vi "S2C_Access_ReadDrvCfg.vi"(8 "Error In":errorcluster) -> (0 "Error Out":errorcluster)   [LabVIEW 2015]
doc: "Reads the data contained within the Settings file and loads the data into VI specific global variables."
uses:
  Core/Command/S2C_CMD_Globals.vi
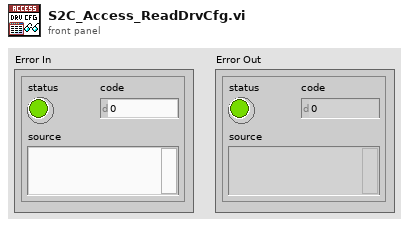
[diagram p1: front panel]
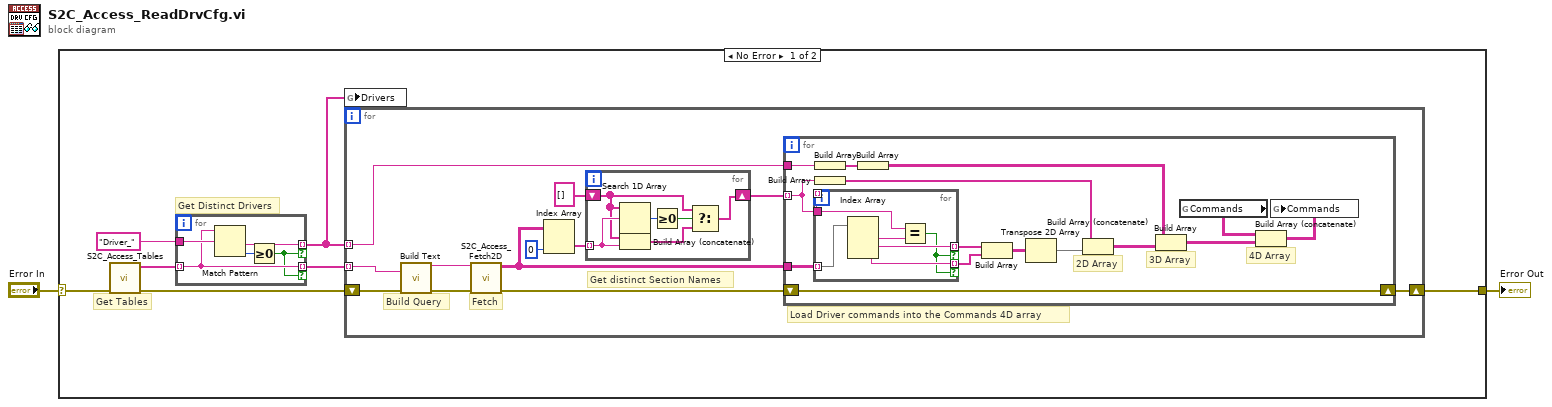
[diagram p0: block diagram]
diagram:
  n1 = case shown="No Error" "Error In" {
    selector: "Error In" -> [w5 w54]
    tunnel: [w4 w54] -> w1
    frame No Error {
      # "Get Distinct Drivers"
      # "Get Tables"
      n2 = call "S2C_Access_Tables.vi"("Error In"=w5) -> ("Error Out"=w7:errorcluster, "Tables"=w9:string[])  [unwired: 9 in]
      n3 = for {
        tunnel: w9 -> [w51] mode=indexing
        tunnel: "Driver_" -> [w53]
        tunnel: [w51] -> w6 mode=indexing if=w49
        tunnel: [w50] -> w3 mode=indexing if=w49
        n4 = Match Pattern(string=w51, regular expression=w53) -> (after substring=w50:string, offset past match=w52:i32)  [unwired: 1 in, 2 out]
        n5 = Greater Or Equal To 0?(x=w52) -> (x >= 0?=w49:bool)
      }
      n6 = global write "S2C_CMD_Globals.vi" "Drivers"(w3) -> ()
      n7 = for {
        shift-right: [w11] -> w4
        shift-left: w7 -> [w21]
        tunnel: w6 -> [w15] mode=indexing
        tunnel: w3 -> [w10] mode=indexing
        # "Load Driver commands into the Commands 4D array"
        # "Get distinct Section Names"
        # "Fetch"
        # "Build Query"
        n8 = call "Build Text"("Driver"=w15, "error in (no error)"=w21) -> ("Result"=w19:string, "error out"=w20:errorcluster)  [unwired: 12 in]
        n9 = call "S2C_Access_Fetch2D.vi"("Error In"=w20, "Query"=w19) -> ("Error Out"=w14:errorcluster, "Data"=w13:string[][])  [unwired: 8 in]
        n10 = Index Array(array=w13, index (col)=0 ("disabled index (col)")) -> (element=w17:string[])  [unwired: 1 in]
        n11 = for {
          shift-right: [w43] -> w12
          shift-left: string[] [] -> [w45]
          tunnel: w17 -> [w46] mode=indexing
          n12 = Search 1D Array(1D array=w45, element=w46) -> (index of element=w48:i32)  [unwired: 1 in]
          n13 = Build Array (concatenate)(w45, w46) -> (w44:string[])
          n14 = Greater Or Equal To 0?(x=w48) -> (x >= 0?=w47:bool)
          n15 = Select(t=w45, s=w47, f=w44) -> (s? t:f=w43:string[])
        }
        n16 = for {
          tunnel: w13 -> [w36]
          shift-right: [w35] -> w11
          shift-left: w14 -> [w35]
          tunnel: w12 -> [w32] mode=indexing
          tunnel: w10 -> [w34]
          # "2D Array"
          # "3D Array"
          # "4D Array"
          n17 = for {
            tunnel: w36 -> [w42] mode=indexing
            tunnel: [w40] -> w31 mode=indexing if=w38
            tunnel: [w39] -> w30 mode=indexing if=w38
            tunnel: w32 -> [w37]
            tunnel: [w37] -> _ mode=indexing
            n18 = Index Array(array=w42) -> (element #1=w41:string, element #2=w40:string, element #3=w39:string)  [unwired: 3 in]
            n19 = Equal?(x=w37, y=w41) -> (x = y?=w38:bool)
          }
          n20 = Build Array(w34) -> (w33:string[])
          n21 = Build Array(w32) -> (w27:string[])
          n22 = Build Array(w33) -> (w25:string[][])
          n23 = Build Array(w31, w30) -> (w29:string[][])
          n24 = Transpose 2D Array(2D array=w29) -> (transposed array=w28:string[][])
          n25 = Build Array (concatenate)(w27, w28) -> (w26:string[][])
          n26 = Build Array(w25, w26) -> (w22:string[][][])
          n27 = global read "S2C_CMD_Globals.vi" "Commands"() -> (w23:string[][][][])
          n28 = Build Array (concatenate)(w23, w22) -> (w24:string[][][][])
          n29 = global write "S2C_CMD_Globals.vi" "Commands"(w24) -> ()
        }
      }
    }
    frame Error {
    }
  }
  "Error Out" <- w1
